vi "AcquirePXIData.vi"(10 "Experiment State":T1={"Send Trigger 3"=FALSE, "error"={"status"=FALSE, "code"=0, "source"=""}, "Digitizer DAQmx Tasks"={"TaskArray"=[]}, "Digitizer Settings"={"6133 Digitizer Channels"=[], "Global Edge Type"=10280, "Total Samples"=[], "Pre-Trigger Samples"=[], "Sample Rate"=[], "Trigger Sources"=[], "Voltage Ranges"=[], "Channel Names"=[], "Active"=[], "Samples to remove"=[], "Start Time"=[], "End Time"=[]}, "Timing Card 2 Fast Outputs"=[{"Delay (s)"=2.559999942779541, "Pulse width (s)"=0.009999999776482582, "Active"=TRUE, "Channel Name"="Fiber 8", "counter"="PXI1Slot8/ctr7"}], "Synchronization Card Settings"={"Position"="PXI1Slot2", "source terminal"="GlobalSoftwareTrigger"}, "Digitizer Data"=[], "Next Shot#"="0", "Timing Card 1 Settings"={"Slot 8 Trigger Source"="", "Clock Source"="", "Trigger Channel Tasks"=[]}, "Timing Card 2 Settings"={"Clock Source"="", "Slot 9 Trigger Source"="", "Trigger Channel Tasks"=[]}, "Timing Card 1 Fast Outputs"=[{"Delay (s)"=2.559999942779541, "Pulse width (s)"=0.009999999776482582, "Active"=TRUE, "Channel Name"="Fiber 8", "counter"="PXI1Slot8/ctr7"}], "System Message"="", "User Shot Notes"=""} {"Timing Card 1 Fast Outputs"."Pulse width (s)" format="%.3p"; "Timing Card 1 Fast Outputs"."Delay (s)" format="%.3p"; "Timing Card 2 Fast Outputs"."Pulse width (s)" format="%.3p"; "Timing Card 2 Fast Outputs"."Delay (s)" format="%.3p"; "Digitizer Settings"."Sample Rate" format="%#_3p"; "Digitizer Settings"."Global Edge Type" items=["Rising"=10280, "Falling"=10171]}) -> (2 "Experiment State":T1={"Send Trigger 3"=FALSE, "error"={"status"=FALSE, "code"=0, "source"=""}, "Digitizer DAQmx Tasks"={"TaskArray"=[]}, "Digitizer Settings"={"6133 Digitizer Channels"=[], "Global Edge Type"=10280, "Total Samples"=[], "Pre-Trigger Samples"=[], "Sample Rate"=[], "Trigger Sources"=[], "Voltage Ranges"=[], "Channel Names"=[], "Active"=[], "Samples to remove"=[], "Start Time"=[], "End Time"=[]}, "Timing Card 2 Fast Outputs"=[{"Delay (s)"=2.559999942779541, "Pulse width (s)"=0.009999999776482582, "Active"=TRUE, "Channel Name"="Fiber 8", "counter"="PXI1Slot8/ctr7"}], "Synchronization Card Settings"={"Position"="PXI1Slot2", "source terminal"="GlobalSoftwareTrigger"}, "Digitizer Data"=[], "Next Shot#"="0", "Timing Card 1 Settings"={"Slot 8 Trigger Source"="", "Clock Source"="", "Trigger Channel Tasks"=[]}, "Timing Card 2 Settings"={"Clock Source"="", "Slot 9 Trigger Source"="", "Trigger Channel Tasks"=[]}, "Timing Card 1 Fast Outputs"=[{"Delay (s)"=2.559999942779541, "Pulse width (s)"=0.009999999776482582, "Active"=TRUE, "Channel Name"="Fiber 8", "counter"="PXI1Slot8/ctr7"}], "System Message"="", "User Shot Notes"=""} {"Timing Card 1 Fast Outputs"."Pulse width (s)" format="%.3p"; "Timing Card 1 Fast Outputs"."Delay (s)" format="%.3p"; "Timing Card 2 Fast Outputs"."Pulse width (s)" format="%.3p"; "Timing Card 2 Fast Outputs"."Delay (s)" format="%.3p"; "Digitizer Settings"."Sample Rate" format="%#_3p"; "Digitizer Settings"."Global Edge Type" items=["Rising"=10280, "Falling"=10171]})   [LabVIEW 2013]
uses:
  <vilib>/Waveform/WDTOps.llb/WDT Get Waveform Time Array DBL.vi
  <vilib>/DAQmx/read.llb/DAQmx Read (Analog 1D Wfm NChan NSamp).vi
  Controls/ExperimentStateCluster.ctl
panel:
  out "data":waveform(dbl)[](array[waveform])
  # "Channel Settings"
  # "Card Wide Settings"
  # "Channel Settings"
  # "Card Wide Settings"
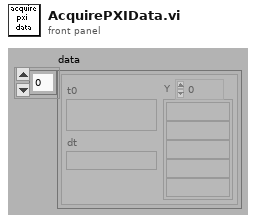
[diagram p1: front panel]
types:
  T1 = typedef "ExperimentStateCluster.ctl" = cluster{"Send Trigger 3":bool, "error":errorcluster, "Digitizer DAQmx Tasks":cluster{"TaskArray":refnum<k21>[]}, "Digitizer Settings":cluster{"6133 Digitizer Channels":tag[][], "Global Edge Type":i32, "Total Samples":i32[], "Pre-Trigger Samples":u32[], "Sample Rate":dbl[], "Trigger Sources":tag[], "Voltage Ranges":dbl[][], "Channel Names":string[][], "Active":bool[][], "Samples to remove":u32[], "Start Time":dbl[], "End Time":dbl[]}, "Timing Card 2 Fast Outputs":cluster{"Delay (s)":dbl, "Pulse width (s)":dbl, "Active":bool, "Channel Name":string, "counter":tag}[], "Synchronization Card Settings":cluster{"Position":refnum<k15>, "source terminal":string}, "Digitizer Data":waveform(dbl)[][], "Next Shot#":string, "Timing Card 1 Settings":cluster{"Slot 8 Trigger Source":tag, "Clock Source":tag, "Trigger Channel Tasks":refnum<k21>[]}, "Timing Card 2 Settings":cluster{"Clock Source":tag, "Slot 9 Trigger Source":tag, "Trigger Channel Tasks":refnum<k21>[]}, "Timing Card 1 Fast Outputs":cluster{"Delay (s)":dbl, "Pulse width (s)":dbl, "Active":bool, "Channel Name":string, "counter":tag}[], "System Message":string, "User Shot Notes":string}
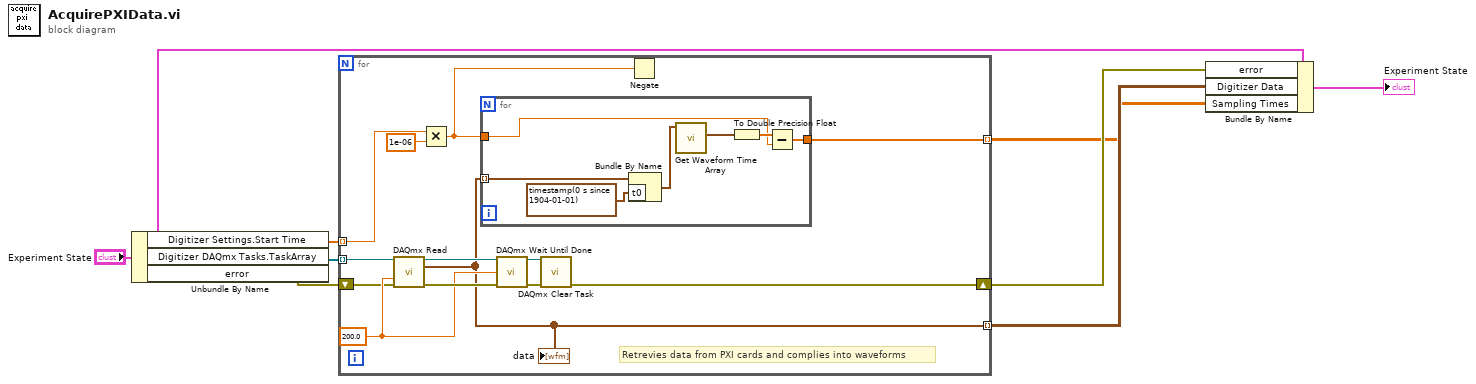
[diagram p0: block diagram]
diagram:
  n1 = Unbundle By Name("Experiment State") -> ("Digitizer Settings.Start Time"=w8:dbl[], "Digitizer DAQmx Tasks.TaskArray"=w7:refnum<k21>[], "error"=w3:errorcluster)
  n2 = for {
    tunnel: w8 -> [w21] mode=indexing
    tunnel: w7 -> [w20] mode=indexing
    tunnel: [w13] -> w4 mode=indexing
    shift-right: [w10] -> w2
    shift-left: w3 -> [w11]
    tunnel: [w9] -> w1 mode=indexing
    w14 = 200.0 ("timeout (sec)")
    # "Retrevies data from PXI cards and complies into waveforms"
    n3 = call-poly <vilib>:"DAQmx Read.vi"("task/channels in"=w20, "timeout"=w14, "error in"=w11) -> ("task out"=w18:refnum<k21>, "data"=w13:waveform(dbl)[], "error out"=w19:errorcluster)  [unwired: 1 in, 9 out]
    "data" <- w13
    n4 = Multiply(x=w21, y=1e-06) -> (x*y=w15:dbl)
    n5 = for {
      tunnel: w13 -> [w23] mode=indexing
      tunnel: [w25] -> w9
      tunnel: w15 -> [w26]
      n6 = Bundle By Name(cluster=w23, "t0"=timestamp(0 s since 1904-01-01)) -> (w22:waveform(dbl))
      n7 = call-poly <vilib>:"Get Waveform Time Array.vi"("waveform in"=w22) -> ("X array"=w28:timestamp[])  [unwired: 1 in, 9 out]
      n8 = To Double Precision Float(number=w28) -> (double precision float=w27:dbl[])
      n9 = Subtract(x=w27, y=w26) -> (x-y=w25:dbl[])
    }
    n10 = call <vilib>:"DAQmx Wait Until Done.vi"("task/channels in"=w18, "timeout (sec)"=w14, "error in"=w19) -> ("task out"=w16:refnum<k21>, "error out"=w17:errorcluster)  [unwired: 11 out]
    n11 = call <vilib>:"DAQmx Clear Task.vi"("task in"=w16, "error in"=w17) -> ("error out"=w10:errorcluster)  [unwired: 13 out]
    n12 = Negate(x=w15) -> ()  [unwired: 1 out]
  }
  n13 = Bundle By Name(cluster="Experiment State", "error"=w2, "Digitizer Data"=w4, "Sampling Times"=w1) -> (→"Experiment State":T1)
